vi "ODE Runge Kutta 4th Order.vi"(0 "time end":dbl=1.0 format="%.2f", 1 "time start":dbl format="%.2f", 2 "h (step rate)":dbl=0.1 min=0.0 format="%.4f", 3 "X0":dbl[](array[numeric]) format="%.2f", 4 "time":string="t", 5 "X (name of variables)":string[](array[string]), 8 "F(X,t) (right sides of the ODE\nas functions of X and t)":string[](array[string])) -> (6 "Times":dbl[](array[numeric]) format="%.2f", 7 "X Values (solution)":dbl[][](array[numeric]) format="%.2f", 9 "ticks":u32, 10 "error":i32)   [LabVIEW 2017, in "NI_Gmath.lvlib"]
doc: "Solves ordinary differential equations with initial conditions using the Runge Kutta method."
uses:
  <vilib>/gmath/NI_Gmath.lvlib
panel:
  out "error message":string
  out "error text":string[](array[string])
  out "error code":i32[](array[numeric])
  # "dX(t)/dt=F(X,t)\nX(0)=X0"
  # "Example:\n\n time start: 0.0 \n time end: 1.0\n h: 0.1\n X0: 1.0 and 1.0 \n time: t\n X: x and y\n F(X,t): sin(t*x)+y and x-y"
  # "further error information"
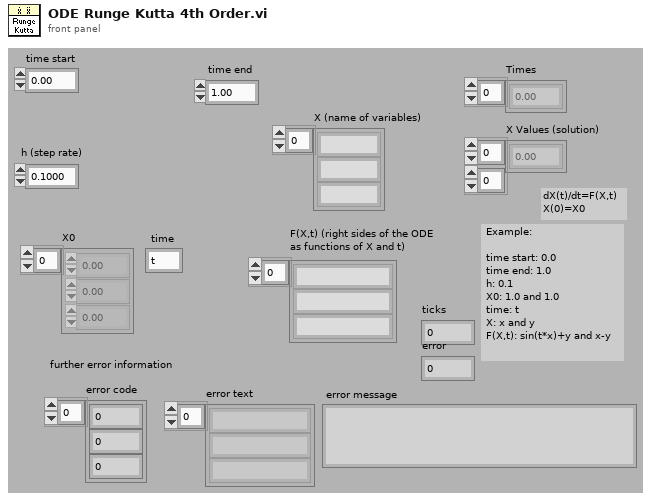
[diagram p1: front panel]
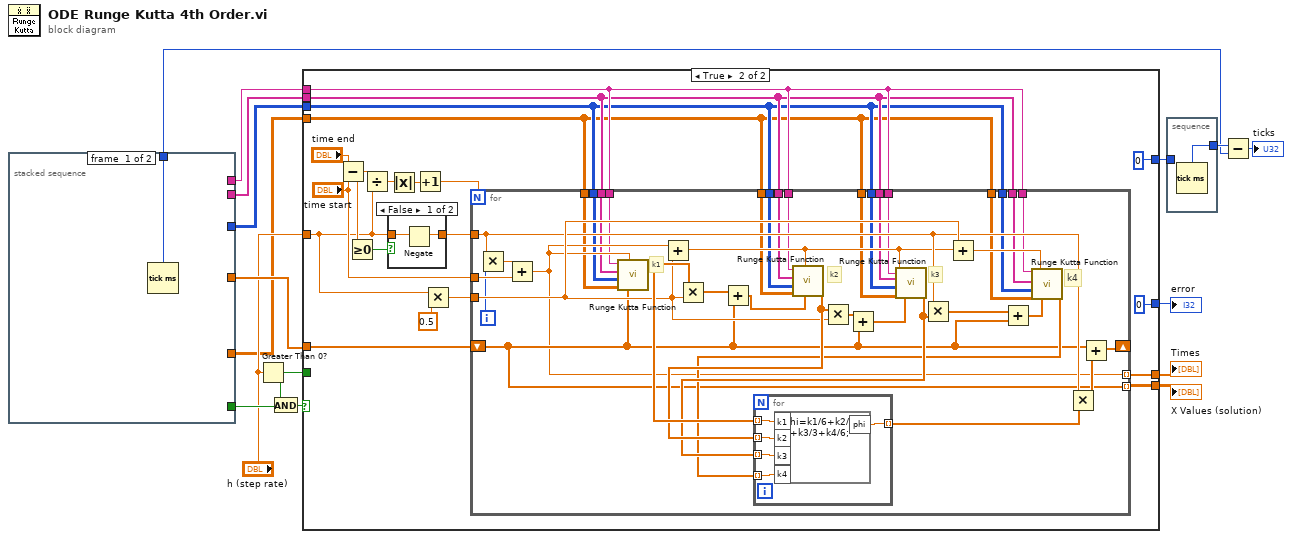
[diagram p0: block diagram]
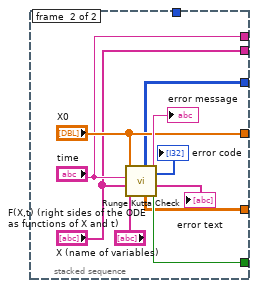
[diagram p2: hidden frame]
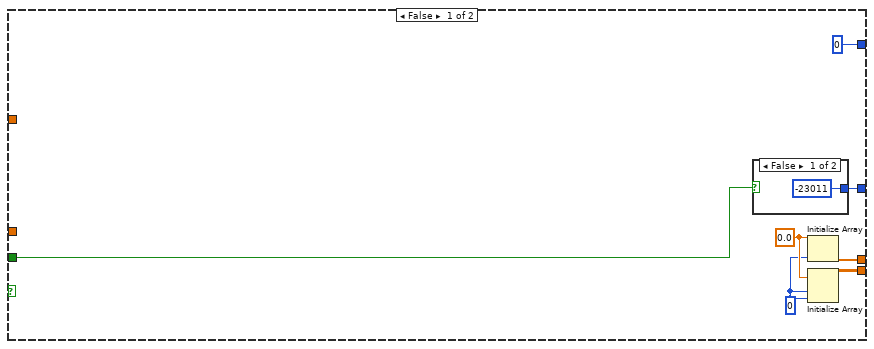
[diagram p3: hidden frame]
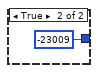
[diagram p4: hidden frame]
diagram:
  n1 = stacked-sequence {
    tunnel: [_ "X0"] -> w14
    tunnel: [_ w27] -> w9
    tunnel: [w17 _] -> w13
    tunnel: [_ w21] -> w2
    tunnel: [_ w20] -> w1
    tunnel: [_ "time"] -> w4
    tunnel: [_ "X (name of variables)"] -> w3
    frame #0 {
      n2 = Tick Count (ms)() -> (millisecond timer value=w17:u32)
    }
    frame #1 {
      n3 = call <vilib>:"Runge Kutta Check.vi"("F(X,t)"="F(X,t) (right sides of the ODE\nas functions of X and t)", "X"="X (name of variables)", "time"="time", "X(0)"="X0") -> ("system OK"=w27:bool, "error text"=→"error text":string[], "error"=→"error code":i32[], "error message"=→"error message":string, "result"=w20:dbl[][], "table"=w21:i32[][][])  [unwired: 2 in]
    }
  }
  n4 = Greater Than 0?(x="h (step rate)") -> (x > 0?=w8:bool)
  n5 = And(x=w8, y=w9) -> (x .and. y?=w7:bool)
  n6 = case shown="True" w7 {
    tunnel: [w31 w47] -> w11
    tunnel: [w32 w50] -> w10
    tunnel: w14 -> [_ w49]
    tunnel: [0 0] -> w12
    tunnel: "h (step rate)" -> [_ w42]
    tunnel: w8 -> [w29 _]
    tunnel: [w28 0] -> w6
    tunnel: w4 -> [_ w40]
    tunnel: w3 -> [_ w39]
    tunnel: w2 -> [_ w38]
    tunnel: w1 -> [_ w37]
    frame False {
      w33 = 0
      w34 = 0.0
      n7 = case shown="False" w29 {
        tunnel: [-23011 -23009] -> w28
        frame False {
        }
        frame True {
        }
      }
      n8 = Initialize Array(w34, w33) -> (w31:dbl[])
      n9 = Initialize Array(w34, w33, w33) -> (w32:dbl[][])
    }
    frame True {
      n10 = Subtract(x="time end", y="time start") -> (x-y=w52:dbl)
      n11 = Greater Or Equal To 0?(x=w52) -> (x >= 0?=w43:bool)
      n12 = Divide(x=w52, y=w42) -> (x/y=w53:dbl)
      n13 = case shown="False" w43 {
        tunnel: [w57 w59] -> w41
        tunnel: w42 -> [w58 w59]
        frame False {
          n14 = Negate(x=w58) -> (-x=w57:dbl)
        }
        frame True {
        }
      }
      n15 = Absolute Value(x=w53) -> (abs(x)=w44:dbl)
      n16 = Increment(x=w44) -> (x+1=w48:dbl)
      n17 = Multiply(x=w42, y=0.5) -> (x*y=w55:dbl)
      n18 = for {
        N: w48 -> [_]
        shift-right: [w84] -> _
        shift-left: w49 -> [w77]
        tunnel: "time start" -> [w97]
        tunnel: w55 -> [w87]
        tunnel: w41 -> [w83]
        tunnel: [w76] -> w47 mode=indexing
        tunnel: [w77] -> w50 mode=indexing
        tunnel: w40 -> [w75]
        tunnel: w39 -> [w74]
        tunnel: w38 -> [w73]
        tunnel: w37 -> [w72]
        tunnel: w40 -> [w71]
        tunnel: w39 -> [w70]
        tunnel: w38 -> [w69]
        tunnel: w37 -> [w68]
        tunnel: w40 -> [w67]
        tunnel: w39 -> [w66]
        tunnel: w38 -> [w65]
        tunnel: w37 -> [w64]
        tunnel: w40 -> [w63]
        tunnel: w39 -> [w62]
        tunnel: w38 -> [w61]
        tunnel: w37 -> [w60]
        i -> [w85]
        # "k4"
        # "k3"
        # "k2"
        # "k1"
        n19 = Multiply(x=w83, y=w85) -> (x*y=w88:dbl)
        n20 = Add(x=w88, y=w97) -> (x+y=w76:dbl)
        n21 = call <vilib>:"Runge Kutta Function.vi"(6:"X"=w77, 7:"time"=w76, "result"=w72, "table"=w73, 10:"X"=w74, 11:"time"=w75) -> ("F(X,time)"=w94:dbl[])  [unwired: 5 in]
        n22 = Add(x=w76, y=w87) -> (x+y=w78:dbl)
        n23 = Multiply(x=w94, y=w87) -> (x*y=w96:dbl[])
        n24 = Add(x=w96, y=w77) -> (x+y=w79:dbl[])
        n25 = call <vilib>:"Runge Kutta Function.vi"(6:"X"=w79, 7:"time"=w78, "result"=w68, "table"=w69, 10:"X"=w70, 11:"time"=w71) -> ("F(X,time)"=w93:dbl[])  [unwired: 5 in]
        n26 = Multiply(x=w93, y=w87) -> (x*y=w95:dbl[])
        n27 = Add(x=w95, y=w77) -> (x+y=w80:dbl[])
        n28 = call <vilib>:"Runge Kutta Function.vi"(6:"X"=w80, 7:"time"=w78, "result"=w64, "table"=w65, 10:"X"=w66, 11:"time"=w67) -> ("F(X,time)"=w92:dbl[])  [unwired: 5 in]
        n29 = Multiply(x=w83, y=w92) -> (x*y=w86:dbl[])
        n30 = Add(x=w87, y=w78) -> (x+y=w81:dbl)
        n31 = Add(x=w86, y=w77) -> (x+y=w82:dbl[])
        n32 = call <vilib>:"Runge Kutta Function.vi"(6:"X"=w82, 7:"time"=w81, "result"=w60, "table"=w61, 10:"X"=w62, 11:"time"=w63) -> ("F(X,time)"=w89:dbl[])  [unwired: 5 in]
        n33 = for {
          tunnel: w89 -> [w102] mode=indexing
          tunnel: [w101] -> w91 mode=indexing
          tunnel: w92 -> [w100] mode=indexing
          tunnel: w93 -> [w99] mode=indexing
          tunnel: w94 -> [w98] mode=indexing
          n34 = formula code="phi=k1/6+k2/3+k3/3+k4/6;"("k1"=w98, "k2"=w99, "k3"=w100, "k4"=w102) -> ("phi"=w101:dbl)
        }
        n35 = Multiply(x=w83, y=w91) -> (x*y=w90:dbl[])
        n36 = Add(x=w77, y=w90) -> (x+y=w84:dbl[])
      }
    }
  }
  "Times" <- w11
  "X Values (solution)" <- w10
  "error" <- w6
  n37 = stacked-sequence {
    tunnel: [w103] -> w16
    tunnel: w12 -> [_]
    frame #0 {
      n38 = Tick Count (ms)() -> (millisecond timer value=w103:u32)
    }
  }
  n39 = Subtract(x=w16, y=w13) -> (x-y=→"ticks":u32)
